vi "Init Device.vi"(7 "Layout Ref":refnum<vi>, 8 "error in (no error)":errorcluster, 10 "Chan# Array":i32[](array[numeric]), 11 "Novatech in":refnum<class "Novatech.lvclass">) -> (0 "error out":errorcluster, 3 "Novatech out":refnum<class "Novatech.lvclass">)   [LabVIEW 2013, in "Novatech.lvclass"]
doc: "Initialize the correct columns and their default appearance. Novatechs always have 4 channels, each requiring three columns so Chan# Array is ignored.\nUse the front panel to change default appearance of the device in the Add/Manage devices."
uses:
  Novatech.lvclass
  ColumnVIs/Column/Column.lvclass
  ColumnVIs/SingleValCol/SingleValCol.lvclass
  TypeDefs/ColumnAppearCluster.ctl
  Novatech.lvclass/Novatech.ctl
panel:
  in  "Default Display":T2(array[cluster])=[{"Channel Name"="", "Columns' Appearance"=[{"Column Name"="", "Width"=30, "Bkgd"=[16448250], "Text"=[0]}, {"Column Name"="", "Width"=30, "Bkgd"=[16448250], "Text"=[0]}, {"Column Name"="", "Width"=30, "Bkgd"=[16448250], "Text"=[0]}]}, {"Channel Name"="", "Columns' Appearance"=[{"Column Name"="", "Width"=30, "Bkgd"=[16448250], "Text"=[0]}, {"Column Name"="", "Width"=30, "Bkgd"=[16448250], "Text"=[0]}, {"Column Name"="", "Width"=30, "Bkgd"=[16448250], "Text"=[0]}]}, {"Channel Name"="", "Columns' Appearance"=[{"Column Name"="", "Width"=30, "Bkgd"=[16448250], "Text"=[0]}, {"Column Name"="", "Width"=30, "Bkgd"=[16448250], "Text"=[0]}, {"Column Name"="", "Width"=30, "Bkgd"=[16448250], "Text"=[0]}]}, {"Channel Name"="", "Columns' Appearance"=[{"Column Name"="", "Width"=30, "Bkgd"=[16448250], "Text"=[0]}, {"Column Name"="", "Width"=30, "Bkgd"=[16448250], "Text"=[0]}, {"Column Name"="", "Width"=30, "Bkgd"=[16448250], "Text"=[0]}]}]
  # "These are the default values that will be presented any\ntime you add a Novatech."
  # "Display Info.vi will automatically append Freq/Amp/Phase to Channel Name (called next!)"
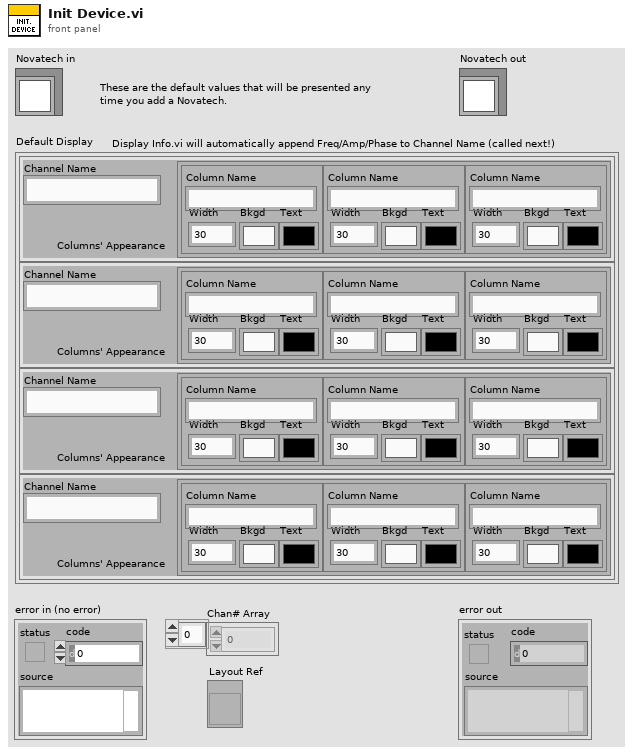
[diagram p1: front panel]
types:
  T1 = typedef "ColumnAppearCluster.ctl" = cluster{"Column Name":string, "Width":u32, "Bkgd":u32[], "Text":u32[]}
  T2 = cluster{"Channel Name":string, "Columns' Appearance":T1[]}[]
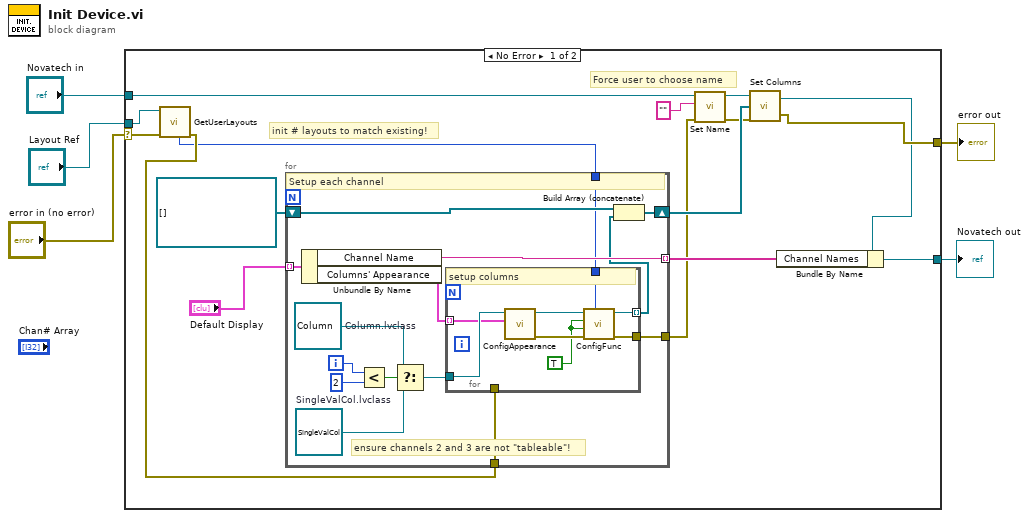
[diagram p0: block diagram]
diagram:
  n1 = case shown="No Error" "error in (no error)" {
    selector: "error in (no error)" -> [w10 w45]
    tunnel: "Novatech in" -> [w17 w46]
    tunnel: [w7 w45] -> w4
    tunnel: [w19 w46] -> w3
    tunnel: "Layout Ref" -> [w11 _]
    frame No Error {
      # "init # layouts to match existing!"
      # "Force user to choose name"
      n2 = call "GetUserLayouts.vi"("error in (no error)"=w10, "Layout Ring Refnum"=w11) -> ("error out"=w9:errorcluster, "Num User Layouts"=w8:i32)  [unwired: 5 in, 3 out]
      n3 = for {
        tunnel: "Default Display" -> [w30] mode=indexing
        tunnel: [w28] -> w18 mode=indexing
        tunnel: w9 -> [w27]
        tunnel: [w26] -> w15
        shift-right: [w23] -> w20
        shift-left: refnum<class "Column.lvclass">[] [] -> [w25]
        tunnel: w8 -> [w22]
        i -> [w33]
        w36 = refnum<class "SingleValCol.lvclass"> refnum  # SingleValCol.lvclass
        w35 = refnum<class "Column.lvclass"> refnum  # Column.lvclass
        # "ensure channels 2 and 3 are not \"tableable\"!"
        # "Setup each channel"
        n4 = Unbundle By Name(w30) -> ("Channel Name"=w28:string, "Columns' Appearance"=w29:T1[])
        n5 = Less?(x=w33, y=2) -> (x < y?=w34:bool)
        n6 = Select(t=w35, s=w34, f=w36) -> (s? t:f=w31:refnum<class "Column.lvclass">)
        n7 = for {
          tunnel: w31 -> [w44]
          tunnel: w29 -> [w43] mode=indexing
          tunnel: w27 -> [_]
          tunnel: [w39] -> w26
          tunnel: [w41] -> w24 mode=indexing
          tunnel: w22 -> [w37]
          w38 = TRUE ("isVariable? (True)")
          # "setup columns"
          n8 = call "ConfigAppearance.vi"("Column Appearance"=w43, "Column in"=w44) -> ("error out"=w40:errorcluster, "Column out"=w42:refnum<class "Column.lvclass">)  [unwired: 8 in]
          n9 = call "ConfigFunc.vi"("Num Layouts (ignored)"=w37, "error in (no error)"=w40, "isVariable? (True)"=w38, "Disableable? (True)"=w38, "Column in"=w42) -> ("error out"=w39:errorcluster, "Column out"=w41:refnum<class "Column.lvclass">)  [unwired: 5 in]
        }
        n10 = Build Array (concatenate)(w25, w24) -> (w23:refnum<class "Column.lvclass">[])
      }
      n11 = call-dynamic "Set Name.vi"("error in (no error)"=w15, "Name"="", "Device in"=w17) -> ("error out"=w14:errorcluster, "Device out"=w16:refnum<class "Novatech.lvclass">)  [unwired: 7 in]
      n12 = call-dynamic "Set Columns.vi"("error in (no error)"=w14, "Columns in"=w20, "Novatech in"=w16) -> ("error out"=w7:errorcluster, "Novatech out"=w6:refnum<class "Novatech.lvclass">)  [unwired: 1 in]
      n13 = Bundle By Name(cluster=w6, "Channel Names"=w18) -> (w19:refnum<class "Novatech.lvclass">)
    }
    frame Error {
    }
  }
  "error out" <- w4
  "Novatech out" <- w3
